vi "Acknowledge Active.vi"(8 "Error In (No Error)":errorcluster, 10 "Sensor Address In":string="a", 11 "RS232 Port In":refnum<visa-resource-name>) -> (0 "Error Out":errorcluster, 2 "Sensor Reply?":bool, 3 "RS232 Port Out":refnum<visa-resource-name>)   [LabVIEW 2015, in "SDI-12.lvlib"]
doc: "Sends an SDI-12 Acknowledge Active command to the specified sensor address. If the sensor replies correctly with a service request, \"Sensor Reply?\" returns true.\n\nSDI-12 Command:\na!\n\nWhere 'a' is a valid address."
uses:
  SDI-12.lvlib
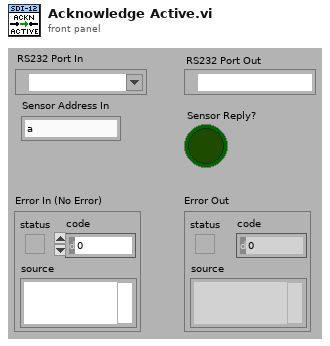
[diagram p1: front panel]
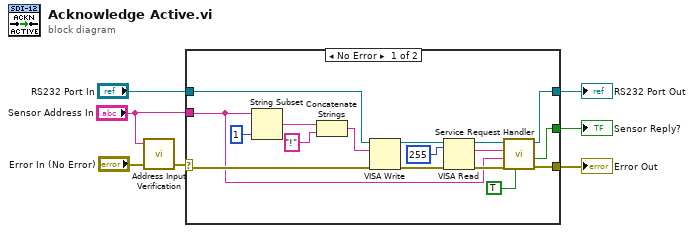
[diagram p0: block diagram]
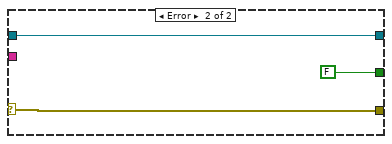
[diagram p2: hidden frame]
diagram:
  n1 = call "Address Input Verification.vi"("Error In (No Error)"="Error In (No Error)", "Sensor Address In (a)"="Sensor Address In") -> ("Error Out"=w5:errorcluster)  [unwired: 2 in, 1 out]
  n2 = case shown="No Error" w5 {
    selector: w5 -> [w18 w27]
    tunnel: [w12 w27] -> w7
    tunnel: "Sensor Address In" -> [w10 _]
    tunnel: [w9 FALSE] -> w3
    tunnel: [w13 w25] -> w2
    tunnel: "RS232 Port In" -> [w11 w25]
    frame No Error {
      n3 = String Subset(string=w10, length (rest)=1 ("length (rest)")) -> (substring=w20:string)  [unwired: 1 in]
      n4 = Concatenate Strings(w20, "!" ("string")) -> (w17:string)
      n5 = VISA Write(VISA resource name=w11, write buffer=w17, error in (no error)=w18) -> (VISA resource name out=w24:refnum<visa-resource-name>, error out=w23:errorcluster)  [unwired: 1 out]
      n6 = VISA Read(VISA resource name=w24, byte count=u32 255, error in (no error)=w23) -> (VISA resource name out=w16:refnum<visa-resource-name>, read buffer=w15:string, error out=w14:errorcluster)  [unwired: 1 out]
      n7 = call "Service Request Handler.vi"("Check address? (False)"=TRUE ("Check address? (false)"), "Error In (No Error)"=w14, "Expected Sensor Address (a)"=w10, "Service Request"=w15, "RS232 Port In"=w16) -> ("Error Out"=w12:errorcluster, "Address Match?"=w9:bool, "RS232 Port Out"=w13:refnum<visa-resource-name>)  [unwired: 3 in, 1 out]
    }
    frame Error {
    }
  }
  "Error Out" <- w7
  "RS232 Port Out" <- w2
  "Sensor Reply?" <- w3
